vi "Measurement UI.vi"() -> ()   [LabVIEW 2021, in "audio_adc_acMeasurementUI.lvlib"]
uses:
  audio_adc_acMeasurementUI.lvlib
panel:
  in  "MeasGraphs":T1(tab)
  out "FreqDomainGraph":cluster{"x0":dbl, "dx":dbl, "magnitude":dbl[]}(graph) caption="AC"
  out "TimeDomainGraph":waveform(dbl)(graph) caption="AC"
  in  "Bit clock edge sync":u32=1
  in  "Frame sync pulse width":u32=32
  in  "Frame length":u32=64
  in  "Data justification":u32 caption="Data Justification"
  in  "Endianness":u32
  in  "Channel 0 offset":u32=1
  in  "Bit depth":u32=24
  in  "Channel length":u32=32
  in  "Channel count per frame":u32=2
  in  "Frame sync edge for channel 0":u32=1
  out "Channel":string
  out "Spectrum":dbl[](array[numeric])
  out "df":dbl
  out "f0":dbl
  out "Time domain":dbl[](array[numeric])
  out "dt":dbl
  out "THD+N":dbl
  out "THD":dbl
  out "SNR":dbl
  out "Calculated amplitude":dbl
  out "Calculated frequency":dbl
  out "SFDR":dbl
  out "Dynamic range":dbl
  out "Gain error":dbl
  out "MeasTable":string[][](table)
  in  "Analog source resource name":string(combo) caption="RESOURCE NAME"
  in  "Configure Protocol Settings":bool
  in  "Protocol capture resource name":string(combo) caption="RESOURCE NAME"
  in  "Channel name":string caption="CHANNEL NAME"
  in  "Channel":u32 caption="CHANNEL"
  in  "Data line":u16 caption="DATA LINE"
  in  "Protocol settings":string="Protocol settings"
  in  "Analog source":string="Analog source "
  in  "Full scale range":dbl=2.825 caption="FULL SCALE RANGE" format="%.3pV"
  in  "Measurement settings":string="Measurement settings"
  in  "MeasSettingsOptions":i32(listbox)=-1
  in  "MeasSettings":bool
  in  "Weighting filter":string(combo)="Linear" caption="WEIGHTING FILTER"
  in  "Measurement duration":dbl=0.1 caption="MEASUREMENT DURATION" format="%#_6ps"
  in  "Sample rate":dbl=44100.0 caption="SAMPLE RATE" format="%#.6pHz"
  in  "Band stop":dbl=20000.0 caption="BAND STOP" format="%#_6pHz"
  in  "Band start":dbl=20.0 caption="BAND START" format="%#_6pHz"
  in  "Amplitude":dbl=-1.0 caption="AMPLITUDE" format="%#_6pdB"
  in  "Frequency":dbl=1000.0 caption="FREQUENCY" format="%#_6pHz"
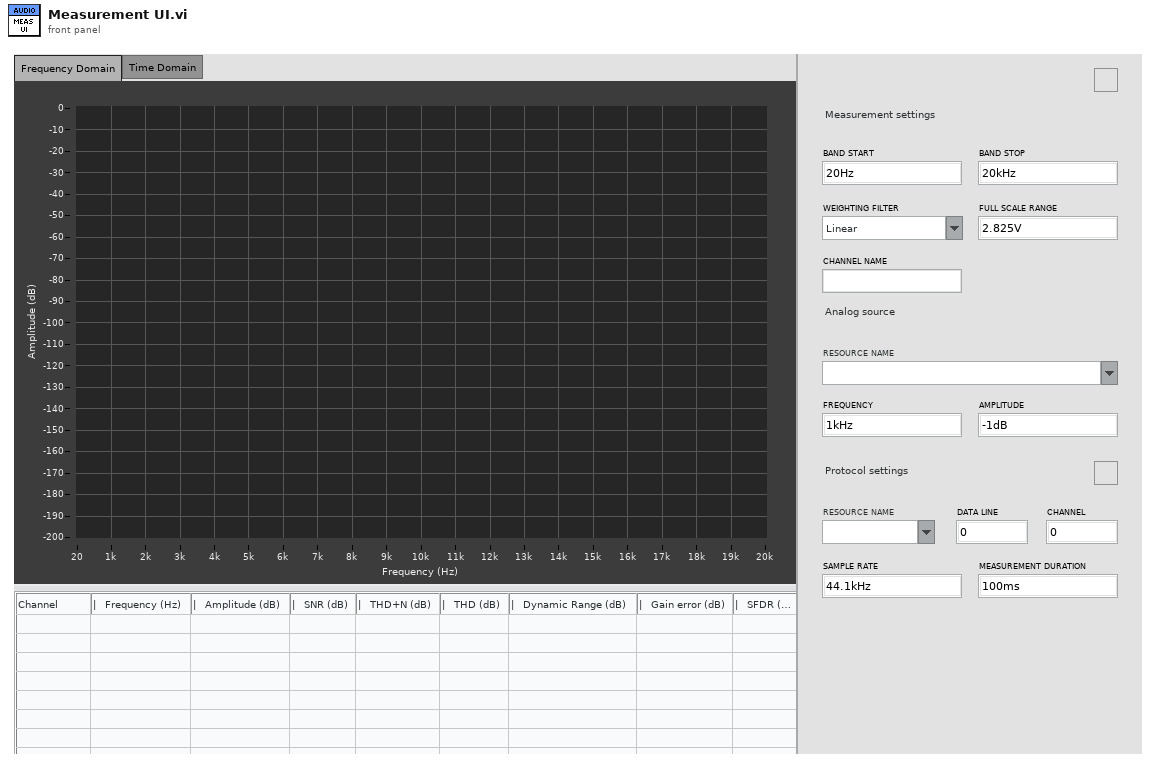
[diagram p1: front panel]
types:
  T1 = enum32{"Frequency Domain", "Time Domain", "Hidden Controls"}
  T2 = enum16{"open", "replace", "create", "open or create", "replace or create", "replace or create with confirmation"}
  T3 = typedef "PDM Shared.lvlib/PCM Frame Sync Control.ctl" = cluster{"Frame Length":u16, "Frame Sync Pulse Width":u16, "Bit Clock Edge  Sync":T4}
  T4 = typedef "PDM Shared.lvlib/Digital Edge.ctl" = enum8{"Rising", "Falling"}
  T5 = typedef "PDM Shared.lvlib/PCM Data Format Configuration.ctl" = cluster{"Frame Sync Edge for Channel 0":T4, "Channel Count Per Frame":u8, "Channel Length":u16, "Bit Depth":u8, "Channel 0 Offset":u16, "Endianness":T6, "Data Justification":T7}
  T6 = typedef "PDM Shared.lvlib/PCM Bit Endianness.ctl" = enum16{"MSB First", "LSB First"}
  T7 = typedef "PDM Shared.lvlib/PCM Data Justification.ctl" = enum16{"Left Justified", "Right Justified"}
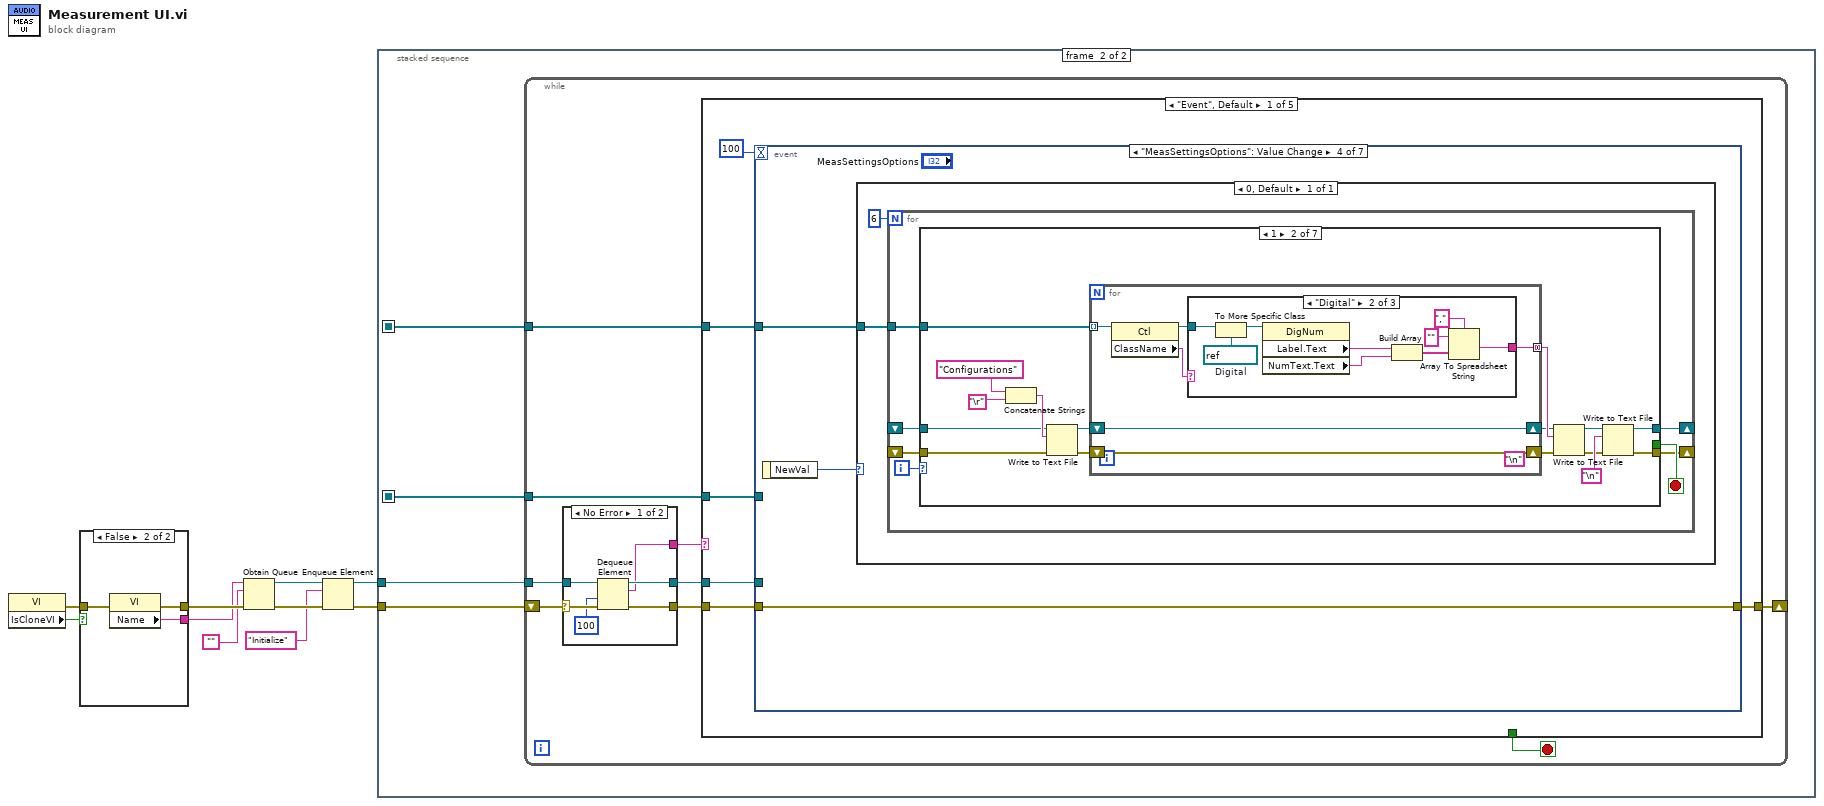
[diagram p0: block diagram]
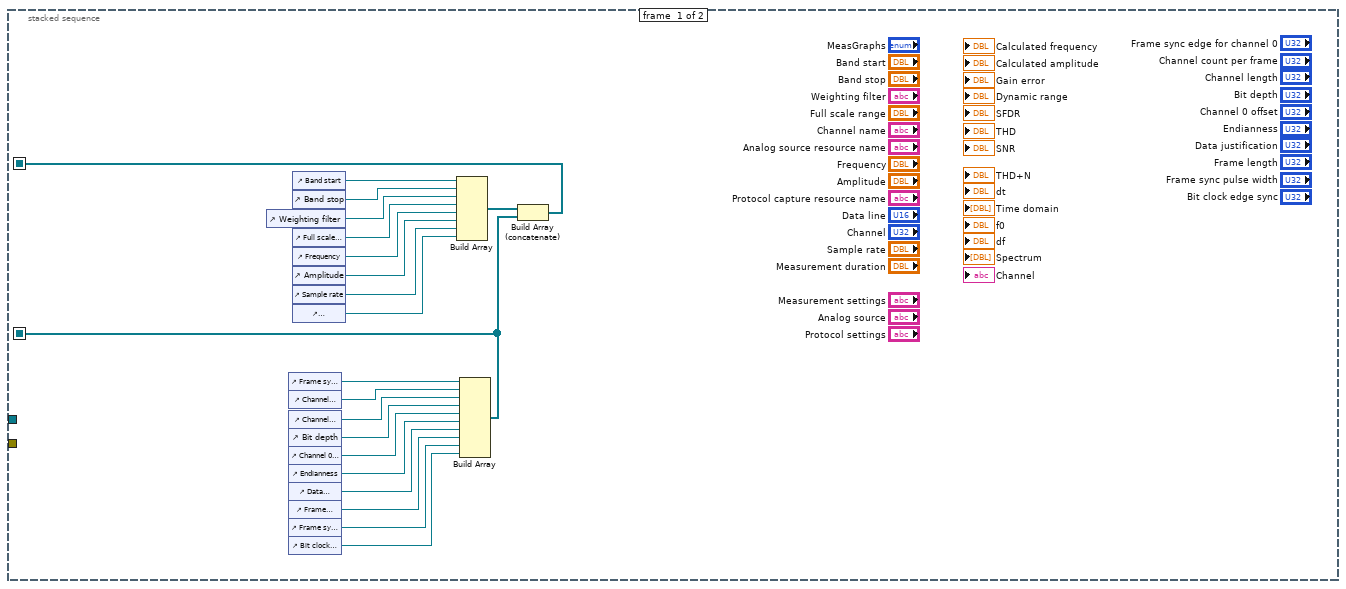
[diagram p2: hidden frame]
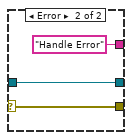
[diagram p3: hidden frame]
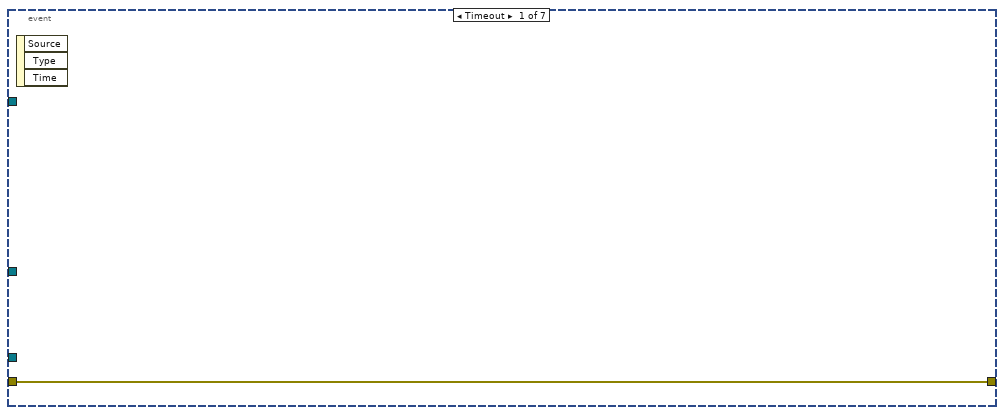
[diagram p4: hidden frame]
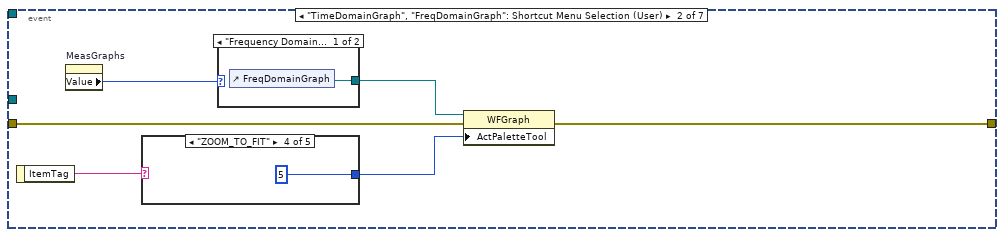
[diagram p5: hidden frame]
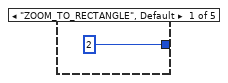
[diagram p6: hidden frame]
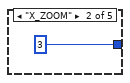
[diagram p7: hidden frame]
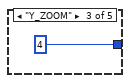
[diagram p8: hidden frame]
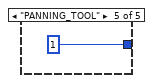
[diagram p9: hidden frame]
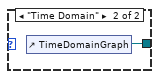
[diagram p10: hidden frame]
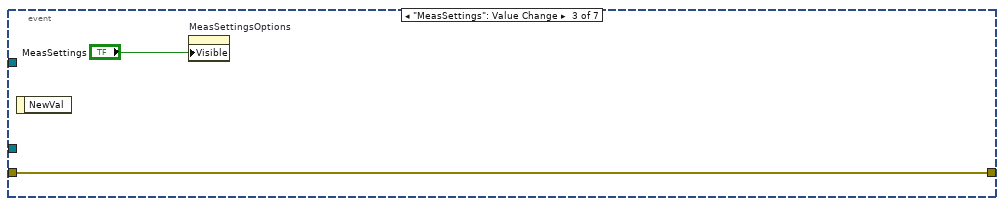
[diagram p11: hidden frame]
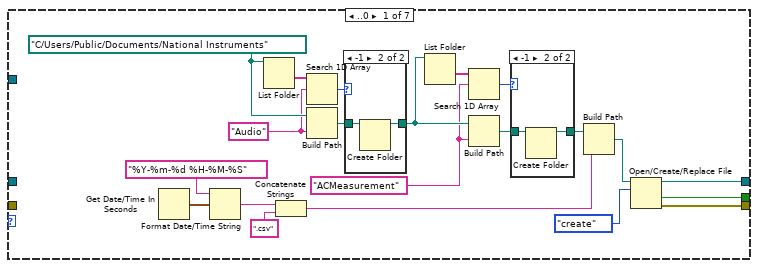
[diagram p12: hidden frame]
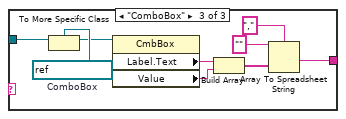
[diagram p16: hidden frame]
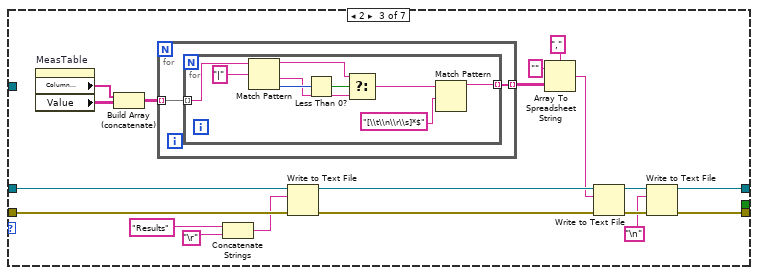
[diagram p17: hidden frame]
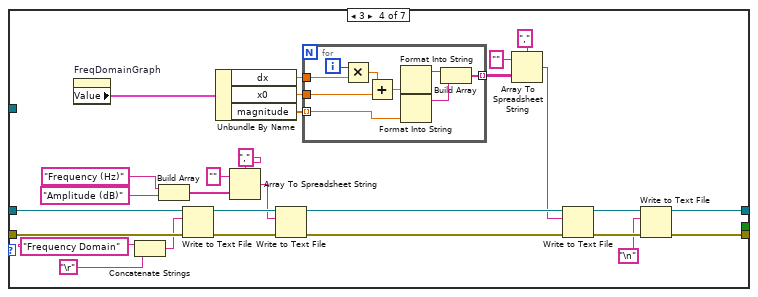
[diagram p18: hidden frame]
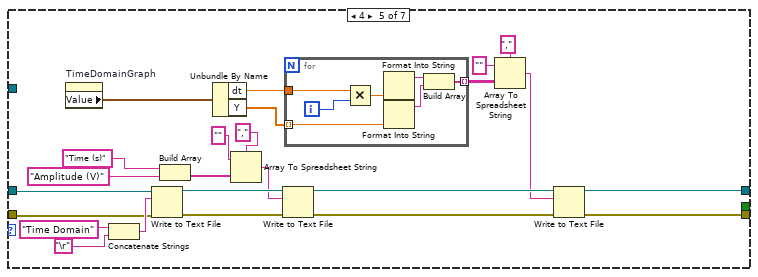
[diagram p19: hidden frame]
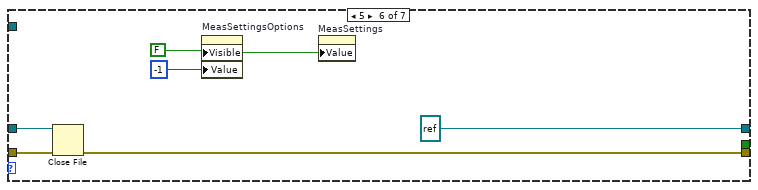
[diagram p20: hidden frame]
diagram:
  n1 = property class="VI"() -> (error out=w1:errorcluster, "IsCloneVI"=w2:bool)  [unwired: 2 in, 1 out]
  n2 = case shown="False" w2 {
    tunnel: [w13 w16] -> w10
    tunnel: [w12 w15] -> w9
    tunnel: w1 -> [w11 w14]
    frame True {
      n3 = property class="VI"(error in=w11) -> (error out=w13:errorcluster, "Clone Name"=w12:string)  [unwired: 1 in, 1 out]
    }
    frame False {
      n4 = property class="VI"(error in=w14) -> (error out=w16:errorcluster, "Name"=w15:string)  [unwired: 1 in, 1 out]
    }
  }
  n5 = Obtain Queue(name (unnamed)=w9, element data type="", error in (no error)=w10) -> (queue out=w6:refnum<queue>, error out=w8:errorcluster)  [unwired: 2 in, 1 out]
  n6 = Enqueue Element(queue=w6, element="Initialize", error in (no error)=w8) -> (queue out=w5:refnum<queue>, error out=w7:errorcluster)  [unwired: 1 in, 1 out]
  n7 = stacked-sequence {
    seq-local: [w17 _] -> [_ w39]
    seq-local: [w19 _] -> [_ w38]
    tunnel: w7 -> [_ w41]
    tunnel: w5 -> [_ w40]
    frame #0 {
      n8 = control-ref of="Weighting filter"() -> (w35:refnum<vi>)
      n9 = control-ref of="Frame sync edge for channel 0"() -> (w29:refnum<vi>)
      n10 = control-ref of="Channel count per frame"() -> (w28:refnum<vi>)
      n11 = control-ref of="Channel length"() -> (w27:refnum<vi>)
      n12 = control-ref of="Bit depth"() -> (w20:refnum<vi>)
      n13 = control-ref of="Channel 0 offset"() -> (w26:refnum<vi>)
      n14 = control-ref of="Endianness"() -> (w25:refnum<vi>)
      n15 = control-ref of="Data justification"() -> (w24:refnum<vi>)
      n16 = control-ref of="Frame length"() -> (w23:refnum<vi>)
      n17 = control-ref of="Frame sync pulse width"() -> (w22:refnum<vi>)
      n18 = control-ref of="Bit clock edge sync"() -> (w21:refnum<vi>)
      n19 = control-ref of="Band start"() -> (w37:refnum<vi>)
      n20 = control-ref of="Band stop"() -> (w36:refnum<vi>)
      n21 = control-ref of="Full scale range"() -> (w34:refnum<vi>)
      n22 = control-ref of="Frequency"() -> (w33:refnum<vi>)
      n23 = control-ref of="Amplitude"() -> (w32:refnum<vi>)
      n24 = control-ref of="Sample rate"() -> (w31:refnum<vi>)
      n25 = control-ref of="Measurement duration"() -> (w30:refnum<vi>)
      n26 = Build Array(w37, w36, w35, w34, w33, w32, w31, w30) -> (w18:refnum<vi>[])
      n27 = Build Array(w29, w28, w27, w20, w26, w25, w24, w23, w22, w21) -> (w19:refnum<vi>[])
      n28 = Build Array (concatenate)(w18, w19) -> (w17:refnum<vi>[])
    }
    frame #1 {
      n29 = while {
        shift-right: [w45] -> _
        shift-left: w41 -> [w50]
        tunnel: w40 -> [w48]
        tunnel: w39 -> [w43]
        tunnel: w38 -> [w42]
        stop <- w44 stop-if-true
        n30 = case shown="No Error" w50 {
          selector: w50 -> [w56 w59]
          tunnel: [w55 w59] -> w49
          tunnel: w48 -> [w54 w58]
          tunnel: [w53 w58] -> w47
          tunnel: [w52 "Handle Error"] -> w46
          frame No Error {
            n31 = Dequeue Element(queue=w54, timeout in ms (-1)=100, error in (no error)=w56) -> (queue out=w53:refnum<queue>, element=w52:string, error out=w55:errorcluster)  [unwired: 1 out]
          }
          frame Error {
          }
        }
        n32 = case shown="\"Event\", Default" w46 {
          tunnel: w49 -> [w64 w283 w327 w342 w343]
          tunnel: w47 -> [w62 _ _ w340 _]
          tunnel: [w65 w283 w327 w337 w343] -> w45
          tunnel: [_ _ _ TRUE _] -> w44
          tunnel: w43 -> [w61 _ _ _ _]
          tunnel: w42 -> [w60 _ _ _ _]
          frame "Event", Default {
            n33 = event shown="[3] \"MeasSettingsOptions\": Value Change" {
              selector: _ -> [_ _ _ _ _ _ _]
              dyn-events: _ -> [_ _ _ _ _ _ _]
              timeout: 100 -> [_ _ _ _ _ _ _]
              tunnel: [w66 w69 _ w84 _ w270 w275] -> w65
              tunnel: w64 -> [w66 w68 w80 w84 _ w270 w276]
              tunnel: w62 -> [_ _ _ _ _ _ w274]
              tunnel: [_ _ w80 _ _ _ _] -> _
              tunnel: w61 -> [_ _ _ w82 _ _ _]
              tunnel: w60 -> [_ _ _ _ w267 _ _]
              event Timeout {
                n34 = event-data() -> ()  [unwired: 1 in, 3 out]
              }
              event "TimeDomainGraph", "FreqDomainGraph": Shortcut Menu Selection (User) {
                n35 = event-data() -> ("ItemTag"=w71:string)  [unwired: 1 in]
                n36 = property on="MeasGraphs" class="TabCtl (strict)"() -> ("Value"=w72:T1)  [unwired: 2 in, 2 out]
                n37 = case shown="\"ZOOM_TO_FIT\"" w71 {
                  tunnel: [2 3 4 5 1] -> w67
                  frame "ZOOM_TO_RECTANGLE", Default {
                  }
                  frame "X_ZOOM" {
                  }
                  frame "Y_ZOOM" {
                  }
                  frame "ZOOM_TO_FIT" {
                  }
                  frame "PANNING_TOOL" {
                  }
                }
                n38 = case shown="\"Frequency Domain\", Default" w72 {
                  tunnel: [w78 w79] -> w70
                  frame "Frequency Domain", Default {
                    n39 = control-ref of="FreqDomainGraph"() -> (w78:refnum<vi>)
                  }
                  frame "Time Domain" {
                    n40 = control-ref of="TimeDomainGraph"() -> (w79:refnum<vi>)
                  }
                }
                n41 = property class="WFGraph"(reference=w70, error in=w68, "ActPaletteTool"=w67) -> (error out=w69:errorcluster)  [unwired: 1 out]
              }
              event "MeasSettings": Value Change {
                n42 = event-data() -> ()  [unwired: 1 in, 1 out]
                n43 = property on="MeasSettingsOptions" class="LstBox (strict)"("Visible"="MeasSettings") -> ()  [unwired: 2 in, 2 out]
              }
              event "MeasSettingsOptions": Value Change {
                n44 = event-data() -> ("NewVal"=w83:i32)  [unwired: 1 in]
                n45 = case shown="0, Default" w83 {
                  tunnel: w82 -> [w85]
                  frame 0, Default {
                    n46 = for {
                      N: 6 -> [_]
                      shift-right: [w91] -> _
                      shift-left: _ -> [w90]
                      shift-right: [w89] -> _
                      shift-left: _ -> [w88]
                      tunnel: w85 -> [w87]
                      i -> [w93]
                      stop <- w92 stop-if-true
                      n47 = case shown="1" w93 {
                        tunnel: [w107 _ _ _ _ _ _] -> w92
                        tunnel: [w113 w121 w168 w195 w236 refnum<file> refnum ("refnum out") w266] -> w91
                        tunnel: w90 -> [_ w132 w179 w218 w237 w264 w266]
                        tunnel: [w106 w123 w167 w193 w235 w262 w265] -> w89
                        tunnel: w88 -> [_ w130 w178 w217 w238 w261 w265]
                        tunnel: w87 -> [_ w133 _ _ _ _ _]
                        frame ..0 {
                          w102 = "ACMeasurement" ("prompt")
                          w109 = "Audio" ("prompt")
                          w112 = path "C:/Users/Public/Documents/National Instruments" ("base path")
                          n48 = Get Date/Time In Seconds() -> (seconds since 1Jan1904=w99:timestamp)
                          n49 = Format Date/Time String(time format string (%c)="%Y-%m-%d %H-%M-%S", seconds (now)=w99) -> (date/time string=w98:string)  [unwired: 1 in]
                          n50 = List Folder(path=w112) -> (folder names=w110:string[])  [unwired: 3 in, 3 out]
                          n51 = Concatenate Strings(w98, ".csv" ("string")) -> (w95:string)
                          n52 = Search 1D Array(1D array=w110, element=w109) -> (index of element=w108:i32)  [unwired: 1 in]
                          n53 = Build Path(base path=w112, name or relative path=w109) -> (appended path=w111:path)
                          n54 = case shown="-1" w108 {
                            tunnel: w111 -> [w118 w120]
                            tunnel: [w118 w119] -> w103
                            frame Default {
                            }
                            frame -1 {
                              n55 = Create Folder(path (use dialog)=w120) -> (created path=w119:path)  [unwired: 2 in, 2 out]
                            }
                          }
                          n56 = List Folder(path=w103) -> (folder names=w105:string[])  [unwired: 3 in, 3 out]
                          n57 = Search 1D Array(1D array=w105, element=w102) -> (index of element=w104:i32)  [unwired: 1 in]
                          n58 = Build Path(base path=w103, name or relative path=w102) -> (appended path=w101:path)
                          n59 = case shown="-1" w104 {
                            tunnel: w101 -> [w115 w117]
                            tunnel: [w115 w116] -> w96
                            frame Default {
                            }
                            frame -1 {
                              n60 = Create Folder(path (use dialog)=w117) -> (created path=w116:path)  [unwired: 2 in, 2 out]
                            }
                          }
                          n61 = Build Path(base path=w96, name or relative path=w95) -> (appended path=w94:path)
                          n62 = Open/Create/Replace File(file path (use dialog)=w94, operation (0:open)=T2."create") -> (refnum out=w113:refnum<file>, cancelled=w107:bool, error out=w106:errorcluster)  [unwired: 4 in]
                        }
                        frame 1 {
                          (unwired) "\n"
                          n63 = Concatenate Strings("Configurations" ("format string"), "\r") -> (w134:string)
                          n64 = Write to Text File(file (use dialog)=w132, text=w134, error in=w130) -> (refnum out=w129:refnum<file>, error out=w131:errorcluster)  [unwired: 1 in, 1 out]
                          n65 = for {
                            tunnel: w133 -> [w138] mode=indexing
                            shift-right: [w142] -> w127
                            shift-left: w129 -> [w142]
                            shift-right: [w141] -> w126
                            shift-left: w131 -> [w141]
                            tunnel: [w140] -> w128 mode=concatenating
                            n66 = property class="Ctl"(reference=w138) -> (reference out=w139:refnum<vi>, "ClassName"=w137:string)  [unwired: 1 in, 1 out]
                            n67 = case shown="\"Digital\"" w137 {
                              tunnel: [_ w146 w156] -> w140
                              tunnel: w139 -> [_ w144 w160]
                              frame Default {
                              }
                              frame "Digital" {
                                w143 = refnum<vi> refnum  # Digital
                                n68 = To More Specific Class(target class=w143, reference=w144) -> (specific class reference=w145:refnum<vi>)  [unwired: 1 in, 1 out]
                                n69 = property class="DigNum"(reference=w145) -> ("Label.Text"=w151:string, "NumText.Text"=w150:string)  [unwired: 1 in, 2 out]
                                n70 = Build Array(w151, w150) -> (w147:string[])
                                n71 = Array To Spreadsheet String(delimiter (Tab)=",", array=w147, 3:"" ("format string")) -> (spreadsheet string=w146:string)
                              }
                              frame "ComboBox" {
                                w159 = refnum<vi> refnum  # ComboBox
                                n72 = To More Specific Class(target class=w159, reference=w160) -> (specific class reference=w155:refnum<vi>)  [unwired: 1 in, 1 out]
                                n73 = property class="CmbBox"(reference=w155) -> ("Label.Text"=w154:string, "Value"=w153:string)  [unwired: 1 in, 2 out]
                                n74 = Build Array(w154, w153) -> (w152:string[])
                                n75 = Array To Spreadsheet String(delimiter (Tab)=",", array=w152, 3:"" ("format string")) -> (spreadsheet string=w156:string)
                              }
                            }
                          }
                          n76 = Write to Text File(file (use dialog)=w127, text=w128, error in=w126) -> (refnum out=w122:refnum<file>, error out=w124:errorcluster)  [unwired: 1 in, 1 out]
                          n77 = Write to Text File(file (use dialog)=w122, text="\n", error in=w124) -> (refnum out=w121:refnum<file>, error out=w123:errorcluster)  [unwired: 1 in, 1 out]
                        }
                        frame 2 {
                          n78 = property on="MeasTable" class="Tbl (strict)"() -> ("Column Headers[]"=w162:string[], "Value"=w161:string[][])  [unwired: 2 in, 2 out]
                          n79 = Build Array (concatenate)(w162, w161) -> (w176:string[][])
                          n80 = for {
                            tunnel: w176 -> [w181] mode=indexing
                            tunnel: [w180] -> w175 mode=indexing
                            n81 = for {
                              tunnel: w181 -> [w183] mode=indexing
                              tunnel: [w182] -> w180 mode=indexing
                              n82 = Match Pattern(string=w183, regular expression="|") -> (before substring=w187:string, after substring=w186:string, offset past match=w189:i32)  [unwired: 1 in, 1 out]
                              n83 = Less Than 0?(x=w189) -> (x < 0?=w188:bool)
                              n84 = Select(t=w187, s=w188, f=w186) -> (s? t:f=w185:string)
                              n85 = Match Pattern(string=w185, regular expression="[\\t\\n\\r\\s]*$") -> (before substring=w182:string)  [unwired: 1 in, 3 out]
                            }
                          }
                          n86 = Concatenate Strings("Results" ("element"), "\r") -> (w163:string)
                          n87 = Write to Text File(file (use dialog)=w179, text=w163, error in=w178) -> (refnum out=w177:refnum<file>, error out=w171:errorcluster)  [unwired: 1 in, 1 out]
                          n88 = Array To Spreadsheet String(delimiter (Tab)=",", array=w175, 3:"" ("format string")) -> (spreadsheet string=w172:string)
                          n89 = Write to Text File(file (use dialog)=w177, text=w172, error in=w171) -> (refnum out=w170:refnum<file>, error out=w169:errorcluster)  [unwired: 1 in, 1 out]
                          n90 = Write to Text File(file (use dialog)=w170, text="\n", error in=w169) -> (refnum out=w168:refnum<file>, error out=w167:errorcluster)  [unwired: 1 in, 1 out]
                        }
                        frame 3 {
                          n91 = property on="FreqDomainGraph" class="WFGraph (strict)"() -> ("Value"=w198:cluster{"x0":dbl, "dx":dbl, "magnitude":dbl[]})  [unwired: 2 in, 2 out]
                          n92 = Concatenate Strings("Frequency Domain" ("string"), "\r") -> (w215:string)
                          n93 = Build Array("Frequency (Hz)", "Amplitude (dB)") -> (w214:string[])
                          n94 = Write to Text File(file (use dialog)=w218, text=w215, error in=w217) -> (refnum out=w211:refnum<file>, error out=w210:errorcluster)  [unwired: 1 in, 1 out]
                          n95 = Unbundle By Name(w198) -> ("dx"=w202:dbl, "x0"=w203:dbl, "magnitude"=w201:dbl[])
                          n96 = Array To Spreadsheet String(delimiter (Tab)=",", array=w214, 3:"" ("format string")) -> (spreadsheet string=w209:string)
                          n97 = Write to Text File(file (use dialog)=w211, text=w209, error in=w210) -> (refnum out=w208:refnum<file>, error out=w207:errorcluster)  [unwired: 1 in, 1 out]
                          n98 = for {
                            tunnel: w201 -> [w222] mode=indexing
                            tunnel: w202 -> [w226]
                            tunnel: w203 -> [w224]
                            tunnel: [w219] -> w204 mode=indexing
                            i -> [w227]
                            n99 = Multiply(x=w227, y=w226) -> (x*y=w225:dbl)
                            n100 = Add(x=w225, y=w224) -> (x+y=w223:dbl)
                            n101 = Format Into String(w223) -> (resulting string=w220:string)  [unwired: 3 in, 1 out]
                            n102 = Format Into String(w222) -> (resulting string=w221:string)  [unwired: 3 in, 1 out]
                            n103 = Build Array(w220, w221) -> (w219:string[])
                          }
                          n104 = Array To Spreadsheet String(delimiter (Tab)=",", array=w204, 3:"" ("format string")) -> (spreadsheet string=w200:string)
                          n105 = Write to Text File(file (use dialog)=w208, text=w200, error in=w207) -> (refnum out=w197:refnum<file>, error out=w196:errorcluster)  [unwired: 1 in, 1 out]
                          n106 = Write to Text File(file (use dialog)=w197, text="\n", error in=w196) -> (refnum out=w195:refnum<file>, error out=w193:errorcluster)  [unwired: 1 in, 1 out]
                        }
                        frame 4 {
                          n107 = property on="TimeDomainGraph" class="WFGraph (strict)"() -> ("Value"=w234:waveform(dbl))  [unwired: 2 in, 2 out]
                          n108 = Concatenate Strings("Time Domain" ("string"), "\r") -> (w250:string)
                          n109 = Write to Text File(file (use dialog)=w237, text=w250, error in=w238) -> (refnum out=w247:refnum<file>, error out=w246:errorcluster)  [unwired: 1 in, 1 out]
                          n110 = Build Array("Time (s)", "Amplitude (V)") -> (w249:string[])
                          n111 = Unbundle By Name(w234) -> ("dt"=w232:dbl, "Y"=w233:dbl[])
                          n112 = Array To Spreadsheet String(delimiter (Tab)=",", array=w249, 3:"" ("format string")) -> (spreadsheet string=w245:string)
                          n113 = Write to Text File(file (use dialog)=w247, text=w245, error in=w246) -> (refnum out=w244:refnum<file>, error out=w243:errorcluster)  [unwired: 1 in, 1 out]
                          n114 = for {
                            tunnel: [w256] -> w240 mode=indexing
                            tunnel: w233 -> [w255] mode=indexing
                            tunnel: w232 -> [w253]
                            i -> [w254]
                            n115 = Multiply(x=w253, y=w254) -> (x*y=w252:dbl)
                            n116 = Format Into String(w252) -> (resulting string=w257:string)  [unwired: 3 in, 1 out]
                            n117 = Format Into String(w255) -> (resulting string=w258:string)  [unwired: 3 in, 1 out]
                            n118 = Build Array(w257, w258) -> (w256:string[])
                          }
                          n119 = Array To Spreadsheet String(delimiter (Tab)=",", array=w240, 3:"" ("format string")) -> (spreadsheet string=w239:string)
                          n120 = Write to Text File(file (use dialog)=w244, text=w239, error in=w243) -> (refnum out=w236:refnum<file>, error out=w235:errorcluster)  [unwired: 1 in, 1 out]
                        }
                        frame 5 {
                          w259 = FALSE ("Visible")
                          n121 = Close File(refnum=w264, error in=w261) -> (error out=w262:errorcluster)  [unwired: 1 out]
                          n122 = property on="MeasSettingsOptions" class="LstBox (strict)"("Visible"=w259, "Value"=-1 ("MeasSettingsOptions")) -> ()  [unwired: 2 in, 2 out]
                          n123 = property on="MeasSettings" class="Bool (strict)"("Value"=w259) -> ()  [unwired: 2 in, 2 out]
                        }
                        frame Default {
                        }
                      }
                    }
                  }
                }
              }
              event "Configure Protocol Settings": Value Change {
                n124 = event-data() -> ()  [unwired: 1 in, 1 out]
                n125 = call "Protocol Settings.vi"() -> ("Frame sync clock control"=w269:T3, "PDM data configuration"=w268:T5)  [unwired: 10 in]
                n126 = call "Update Protocol UI Controls.vi"("Frame Sync Clock Control"=w269, "PCM Data Configuration"=w268, "Control references"=w267) -> ()  [unwired: 9 in]
              }
              event Mouse Down {
                w271 = FALSE ("Visible")
                n127 = event-data() -> ()  [unwired: 1 in, 1 out]
                n128 = property on="MeasSettingsOptions" class="LstBox (strict)"("Visible"=w271, "Value"=-1 ("MeasSettingsOptions")) -> ()  [unwired: 2 in, 2 out]
                n129 = property on="MeasSettings" class="Bool (strict)"("Value"=w271) -> ()  [unwired: 2 in, 2 out]
              }
              event Panel Close? {
                n130 = event-data() -> ()  [unwired: 1 in, 4 out]
                n131 = Enqueue Element(queue=w274, element="Exit", error in (no error)=w276) -> (error out=w275:errorcluster)  [unwired: 1 in, 2 out]
                n132 = event-data("Discard?"=TRUE) -> ()  [unwired: 1 in, 1 out]
              }
            }
          }
          frame "Initialize" {
            w281 = string[] ["Export data"] ("Item Names")
            n133 = for {
              N: 2 -> [_]
              i -> [w292]
              n134 = case shown="1" w292 {
                tunnel: [w295 w296] -> w293
                frame 0, Default {
                  n135 = control-ref of="FreqDomainGraph"() -> (w295:refnum<vi>)
                }
                frame 1 {
                  n136 = control-ref of="TimeDomainGraph"() -> (w296:refnum<vi>)
                }
              }
              n137 = property class="WFGraph"(reference=w293, "ActPaletteTool"=2 ("Palette:Active Tool")) -> ()  [unwired: 1 in, 2 out]
            }
            n138 = property on="MeasSettingsOptions" class="LstBox (strict)"("Item Names"=w281, "Value"=-1 ("MeasSettingsOptions"), "Visible"=FALSE, "Disabled Items"=i32[] []) -> ()  [unwired: 2 in, 2 out]
            n139 = for {
              tunnel: w281 -> [_] mode=indexing
              i -> [w291]
              n140 = property on="MeasSettingsOptions" class="LstBox (strict)"("Active Row"=w291, "Cell Height"=30 ("Active Row:Cell Height")) -> ()  [unwired: 2 in, 2 out]
            }
            n141 = stacked-sequence {
              frame #0 {
                n142 = call "Detected DSGs.vi"() -> ("AO channels"=w286:string[])  [unwired: 11 in]
                n143 = Index Array(array=w286, index=0) -> (element=w285:string)
                n144 = property on="Analog source resource name" class="CmbBox"("Strings[]"=w286, "Value"=w285) -> ()  [unwired: 2 in, 2 out]
              }
              frame #1 {
                n145 = call "Detected PDMs.vi"() -> ("PDM devices"=w289:string[])  [unwired: 11 in]
                n146 = Index Array(array=w289, index=0) -> (element=w288:string)
                n147 = property on="Protocol capture resource name" class="CmbBox"("Strings[]"=w289, "Value"=w288) -> ()  [unwired: 2 in, 2 out]
              }
            }
          }
          frame "Post UI Update" {
            w309 = "|   " ("initial string")
            # "This case will be triggered, after framework updates the User interface with result values."
            n148 = local read "Time domain"() -> (w326:dbl[])
            n149 = local read "Spectrum"() -> (w300:dbl[])
            n150 = local read "df"() -> (w302:dbl)
            n151 = local read "dt"() -> (w325:dbl)
            n152 = local read "f0"() -> (w299:dbl)
            n153 = local read "Calculated frequency"() -> (w312:dbl)
            n154 = local read "Calculated amplitude"() -> (w311:dbl)
            n155 = local read "Dynamic range"() -> (w321:dbl)
            n156 = Bundle By Name("Y"=w326, "dt"=w325) -> (→"TimeDomainGraph":waveform(dbl))  [unwired: 1 in]
            n157 = Bundle(cluster=cluster{"x0":dbl, "dx":dbl, "magnitude":dbl[]} {"x0"=0.0, "dx"=0.0, "magnitude"=[]} ("FreqDomainGraph"), "x0"=w299, "dx"=w302, "magnitude"=w300) -> (→"FreqDomainGraph":cluster{"x0":dbl, "dx":dbl, "magnitude":dbl[]})
            n158 = local read "THD+N"() -> (w322:dbl)
            n159 = local read "Gain error"() -> (w308:dbl)
            n160 = local read "THD"() -> (w323:dbl)
            n161 = local read "SNR"() -> (w310:dbl)
            n162 = local read "SFDR"() -> (w307:dbl)
            n163 = Build Array(w312, w311) -> (w318:dbl[])
            n164 = Build Array(w310, w322, w323, w321) -> (w317:dbl[])
            n165 = for {
              tunnel: w318 -> [w332] mode=indexing
              tunnel: w309 -> [w333]
              tunnel: "%.3f" ("initial string") -> [w334]
              tunnel: [w335] -> w316 mode=indexing
              n166 = Format Into String(format string=w334, initial string=w333, w332) -> (resulting string=w335:string)  [unwired: 1 in, 1 out]
            }
            n167 = for {
              tunnel: w317 -> [w328] mode=indexing
              tunnel: w309 -> [w329]
              tunnel: "%5.1f" ("initial string") -> [w330]
              tunnel: [w331] -> w315 mode=indexing
              n168 = Format Into String(format string=w330, initial string=w329, w328) -> (resulting string=w331:string)  [unwired: 1 in, 1 out]
            }
            n169 = Format Into String(format string="%5.1f" ("initial string"), initial string=w309, w307) -> (resulting string=w305:string)  [unwired: 1 in, 1 out]
            n170 = Format Into String(format string="%5.3f" ("initial string"), initial string=w309, w308) -> (resulting string=w306:string)  [unwired: 1 in, 1 out]
            n171 = local read "Channel"() -> (w297:string)
            n172 = Build Array (concatenate)(w297, w316, w315, w306, w305) -> (w314:string[])
            n173 = Build Array(w314) -> (→"MeasTable":string[][])
          }
          frame "Exit" {
            # "This case is triggered to close the User Interface from framework"
            n174 = Flush Queue(queue=w340, error in (no error)=w342) -> (queue out=w339:refnum<queue>, error out=w338:errorcluster)  [unwired: 1 out]
            n175 = Release Queue(queue=w339, force destroy? (F)=TRUE, error in (no error)=w338) -> (error out=w337:errorcluster)  [unwired: 2 out]
          }
          frame "Handle Error" {
          }
        }
      }
    }
  }
